vi "3st body.vi"(0 "third test item name":string, 1 "file path (dialog if empty)":path caption="文件路径 （空时为对话框）", 2 "ABS?":bool, 3 "Points":dbl[](array[numeric]), 5 "second result":string, 7 "single spec":dbl[](array[numeric]), 9 "TDD spec":string, 11 "SN":string, 12 "limit type":enum16{"上限", "下限"}(ring), 13 "TDD?":bool) -> (6 "OutPutXml":string)   [LabVIEW 2011]
panel:
  out "pointValue":string[][](array[string])
  out "all rows":string[][](array[string])
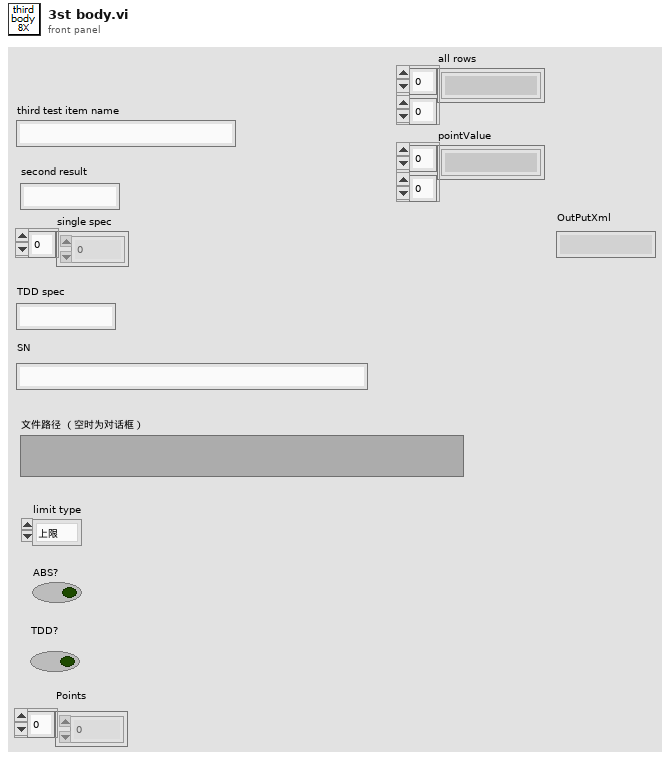
[diagram p1: front panel]
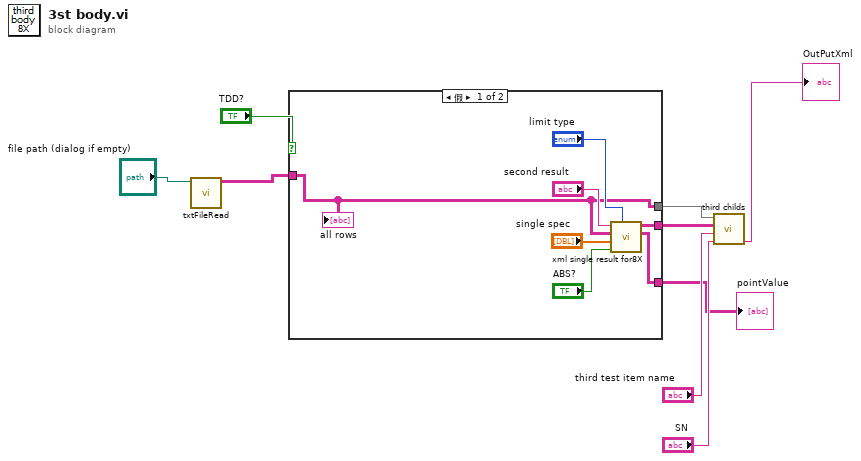
[diagram p0: block diagram]
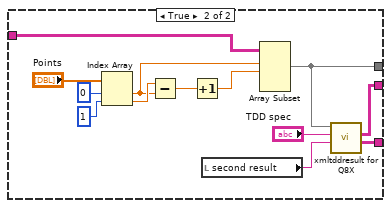
[diagram p2: hidden frame]
diagram:
  n1 = call "txtFileRead.vi"("file path (dialog if empty)"="file path (dialog if empty)") -> ("all rows"=w2:string[][])  [unwired: 10 in]
  n2 = case shown="假" "TDD?" {
    tunnel: w2 -> [w14 w29]
    tunnel: [w14 w21] -> w5
    tunnel: [w11 w18] -> w8
    tunnel: [w10 w17] -> w1
    frame False {
      n3 = call "xml single result for8X.vi"("limitType"="limit type", "abs?"="ABS?", "single spec"="single spec", "dataSource"=w14, "second result"="second result") -> ("pointValue"=w10:string[][], "third result"=w11:string[][])  [unwired: 5 in]
      "all rows" <- w14
    }
    frame True {
      n4 = Index Array(array="Points", index #1=0 ("索引"), index #2=1 ("索引")) -> (element #1=w24:dbl, element #2=w25:dbl)
      n5 = Subtract(x=w25, y=w24) -> (x-y=w23:dbl)
      n6 = Increment(x=w23) -> (x+1=w22:dbl)
      n7 = local read "second result"() -> (w19:string)
      n8 = Array Subset(array=w29, index (row)=w24, length (row)=w22) -> (w21:string[][])  [unwired: 2 in]
      n9 = call "xmltddresult for Q8X.vi"("second result"=w19, "TDD spec"="TDD spec", "TDD array"=w21) -> ("pointValue"=w17:string[][], "TDD third result"=w18:string[][])  [unwired: 7 in]
    }
  }
  "pointValue" <- w1
  n10 = call "third childs.vi"("SN"="SN", "third test item name"="third test item name", "third result"=w8, "all rows"=w5) -> ("thirdChilds"=→"OutPutXml":string)  [unwired: 7 in]
